vi "8.1.vi"() -> ()   [LabVIEW 2017]
panel:
  out "Numeric":dbl
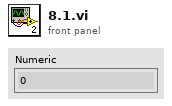
[diagram p1: front panel]
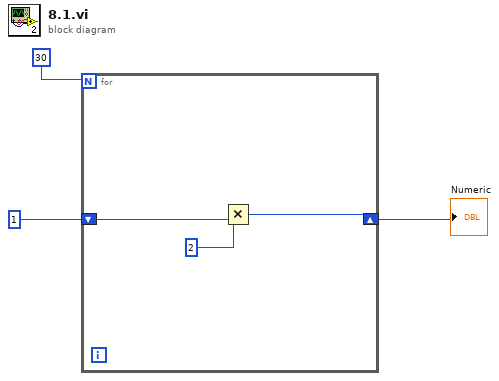
[diagram p0: block diagram]
diagram:
  n1 = for {
    N: 30 -> [_]
    shift-right: [w4] -> w1
    shift-left: 1 -> [w6]
    n2 = Multiply(x=w6, y=2) -> (x*y=w4:i32)
  }
  "Numeric" <- w1
